vi "On Compile - Parse System Definition and Initialize Data Refs.vi"(8 "error in":errorcluster, 11 "custom device ref in":T1 format="%.0x") -> (0 "error out":errorcluster)   [LabVIEW 2020, in "Ballard ARINC 429 System Explorer.lvlib"]
uses:
  Ballard ARINC 429 System Explorer.lvlib
  Shared/Ballard ARINC 429 Shared.lvlib
  Shared/Direction.ctl
  <vilib>/NI VeriStand/Custom Device API/Custom Device API.lvlib
  Shared/Label.ctl
  Encoding and Decoding/Encoding.ctl
  Encoding and Decoding/Encoding and Decoding.lvlib
  Protocol/Implementations/ARINC429/Parameter Definition.ctl
  Protocol/Implementations/ARINC429/ARINC 429.lvclass
  <vilib>/NI VeriStand/Custom Device API/Data Reference.ctl
  <vilib>/NI VeriStand/Custom Device API/Block Data Reference.ctl
  <vilib>/NI VeriStand/Custom Device API/Custom Device Item Ref.ctl
  Shared/RT Parameters.ctl
  Shared/Transfer Type.ctl
  Shared/RT Label Settings.ctl
  Shared/RT Hardware Channel Settings.ctl
  <vilib>/NI/NIVS Inline Async API/_Data Access System Explorer/Data Access System Explorer.lvlib
  Shared/Constants.vi
  <vilib>/NI VeriStand/Custom Device API/Set Item Property (Variant).vi
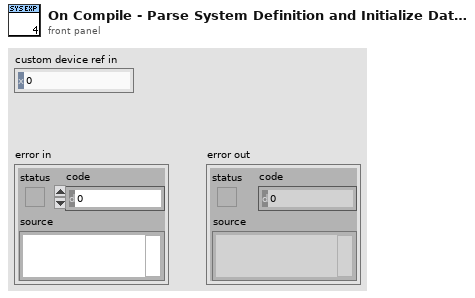
[diagram p1: front panel]
types:
  T1 = typedef "Custom Device API.lvlib/Custom Device Item Ref.ctl" = u64
  T2 = typedef "Ballard ARINC 429 Shared.lvlib/RT Hardware Channel Settings.ctl" = cluster{"channel #":u16, "channel handle":u64, "labels settings for RT":T3[]}
  T3 = typedef "Ballard ARINC 429 Shared.lvlib/RT Label Settings.ctl" = cluster{"Name":string, "xmlName":string, "label":T4, "transfer period":u32, "SDI_Enabled":bool, "SDI":u8, "parameter driver data":T5, "transfer type":T10, "has timestamp?":bool, "Label Disable/Trigger Channel Reference":T1, "Message Handle":u64, "Initialized?":bool, "Word Initial Raw Value":u32, "Label Timestamp Channel Data Reference":T9}
  T4 = typedef "Ballard ARINC 429 Shared.lvlib/Label.ctl" = u8
  T5 = typedef "Ballard ARINC 429 Shared.lvlib/RT Parameters.ctl" = cluster{"parameter definitions":T6[], "Rx block data refs":T8[], "Rx values":dbl[], "Tx parameter refs":T1[]}
  T6 = typedef "ARINC 429.lvclass/Parameter Definition.ctl" = cluster{"start index":i32, "size":i32, "encoding":T7, "signed":bool, "scale multiplier":dbl, "scale offset":dbl}
  T7 = typedef "Encoding and Decoding.lvlib/Encoding.ctl" = enum16{"BNR", "BCD", "Discrete"}
  T8 = typedef "Custom Device API.lvlib/Block Data Reference.ctl" = cluster{"Data Reference":T9, "Offset":u64, "Length":u64}
  T9 = typedef "Custom Device API.lvlib/Data Reference.ctl" = i32
  T10 = typedef "Ballard ARINC 429 Shared.lvlib/Transfer Type.ctl" = enum16{"Scheduled", "Acyclic", "Block", "Strobe"}
  T11 = cluster{"Name":string, "Rx configuration":T2[], "Tx configuration":T2[]}
  T12 = typedef "Ballard ARINC 429 Shared.lvlib/Direction.ctl" = enum16{"Rx", "Tx"}
  T13 = typedef "Custom Device API.lvlib/Custom Device Item Info.ctl" = cluster{"Name":string, "Is Channel":bool, "GUID":string, "Is Waveform":bool}
  T14 = cluster{"Name":string, "Type":enum16{"Output/Write", "Input/Read", "Input/ReadWrite"}, "VS Refs":T1[]}
  T15 = cluster{"Name":string, "Type":enum16{"Output/Write", "Input/Read", "Input/ReadWrite"}, "VS Refs":T1[]}[]
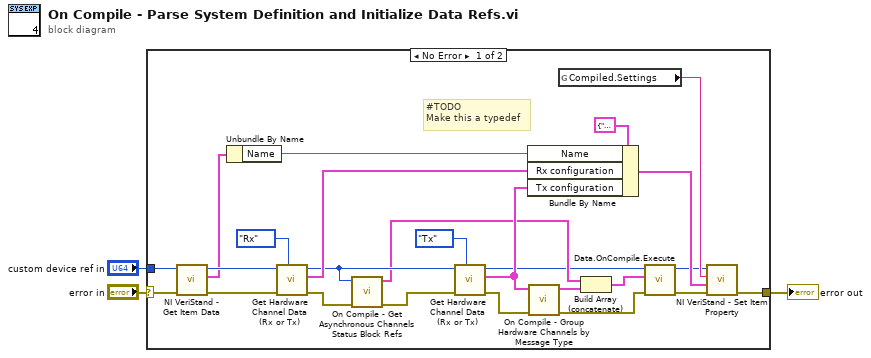
[diagram p0: block diagram]
diagram:
  n1 = case shown="No Error" "error in" {
    selector: "error in" -> [w15 w29]
    tunnel: "custom device ref in" -> [w26 _]
    tunnel: [w14 w29] -> w1
    frame No Error {
      # "#TODO\nMake this a typedef"
      n2 = call <vilib>:"NI VeriStand - Get Item Data.vi"("error in (no error)"=w15, "Item Ref in"=w26) -> ("error out"=w24:errorcluster, "Item Info"=w23:T13, "Item Ref out"=w25:T1)  [unwired: 6 in, 1 out]
      n3 = Unbundle By Name(w23) -> ("Name"=w22:string)
      n4 = call "Get Hardware Channel Data (Rx or Tx).vi"("direction"=Direction."Rx", "error in"=w24, "custom device ref in"=w25) -> ("error out"=w12:errorcluster, "hardware channel data"=w21:T2[], "custom device ref out"=w13:T1)  [unwired: 6 in]
      n5 = call "On Compile - Get Asynchronous Channels Status Block Refs.vi"("error in"=w12, "Item Ref"=w13) -> ("error out"=w11:errorcluster, "Async Status Channels Refs"=w5:T14)  [unwired: 8 in]
      n6 = call "Get Hardware Channel Data (Rx or Tx).vi"("direction"=Direction."Tx", "error in"=w11, "custom device ref in"=w13) -> ("error out"=w7:errorcluster, "hardware channel data"=w9:T2[], "custom device ref out"=w4:T1)  [unwired: 6 in]
      n7 = Bundle By Name(cluster=T11 {"Name"="", "Rx configuration"=[], "Tx configuration"=[]}, "Name"=w22, "Rx configuration"=w21, "Tx configuration"=w9) -> (w18:T11)
      n8 = call "On Compile - Group Hardware Channels by Message Type.vi"("error in"=w7, "hardware channel data"=w9) -> ("error out"=w6:errorcluster, "grouped hardware channel data refs"=w8:T15)  [unwired: 8 in]
      n9 = global read "Constants.vi" "Compiled.Settings"() -> (w19:string)
      n10 = Build Array (concatenate)(w5, w8) -> (w10:T15)
      n11 = call <vilib>:"Data.OnCompile.Execute.vi"("error in"=w6, "VS Ref Groups"=w10, "Custom Device Ref"=w4) -> ("error out"=w16:errorcluster, "Custom Device Ref"=w17:T1)  [unwired: 7 in]
      n12 = call-poly <vilib>:"NI VeriStand - Set Item Property.vi"("error in (no error)"=w16, "Value"=w18, "Property Name"=w19, "Item Ref in"=w17) -> ("error out"=w14:errorcluster)  [unwired: 5 in, 2 out]
    }
    frame Error {
    }
  }
  "error out" <- w1
